vi "rx.vi"() -> ()   [LabVIEW 2020]
panel:
  out "array":i32[](array[numeric])
  out "read buffer":string
  in  "Serial Init":T1={"Puerto Serial"="", "baud rate (9600)"=9600, "data bits (8)"=8, "parity (0:none)"=enum."None", "error in (no error)"={"status"=FALSE, "code"=0, "source"=""}, "stop bits (10: 1 bit)"=10, "flow control (0:none)"=0} {"flow control (0:none)" items=["None", "XON/XOFF", "RTS/CTS", "XON/XOFF & RTS/CTS", "DTR/DSR", "XON/XOFF & DTR/DSR"]; "stop bits (10: 1 bit)" items=["1.0"=10, "1.5"=15, "2.0"=20]; "data bits (8)" min=5 max=8 step=1}
  in  "stop":bool
  # "Recepcion Serial"
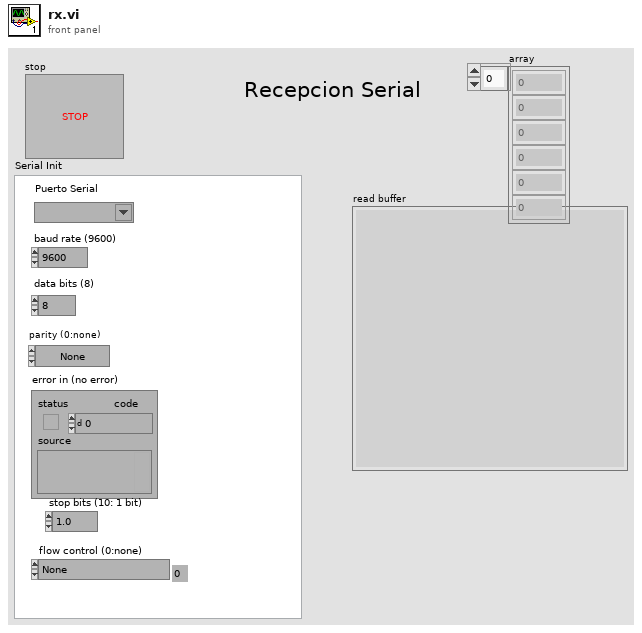
[diagram p1: front panel]
types:
  T1 = cluster{"Puerto Serial":refnum<visa-resource-name>, "baud rate (9600)":u32, "data bits (8)":u16, "parity (0:none)":enum16{"None", "Odd", "Even", "Mark", "Space"}, "error in (no error)":errorcluster, "stop bits (10: 1 bit)":u16, "flow control (0:none)":u16}
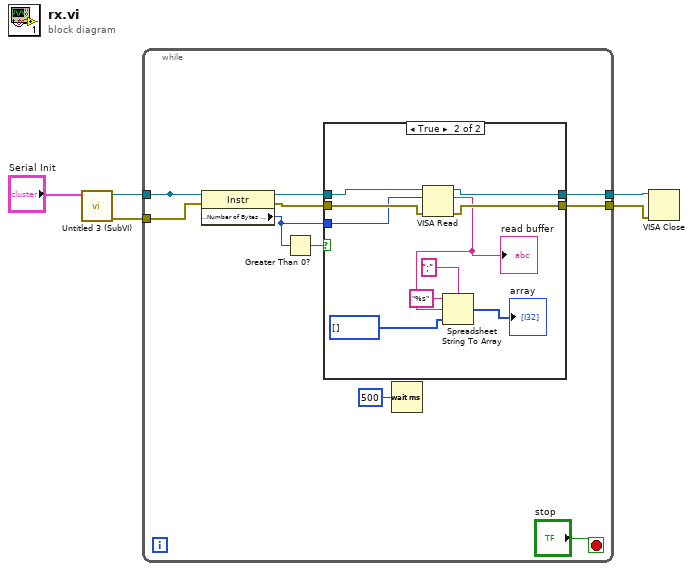
[diagram p0: block diagram]
diagram:
  n1 = call "Untitled 3 (SubVI).vi"("Serial Init"="Serial Init") -> ("error out"=w3:errorcluster, "VISA Refnum out"=w4:refnum<visa-resource-name>)  [unwired: 9 in]
  n2 = while {
    tunnel: [w14] -> _
    tunnel: w4 -> [w14]
    tunnel: w3 -> [w13]
    tunnel: [w10] -> w2
    tunnel: [w8] -> w1
    stop <- "stop" stop-if-true
    n3 = property class="Instr"(reference=w14, error in=w13) -> (reference out=w9:refnum<visa-resource-name>, error out=w7:errorcluster, "Serial Settings:Number of Bytes at Serial Port"=w6:u32)
    n4 = Greater Than 0?(x=w6) -> (x > 0?=w11:bool)
    n5 = case shown="True" w11 {
      tunnel: [w17 w24] -> w10
      tunnel: w9 -> [w17 w27]
      tunnel: [w16 w23] -> w8
      tunnel: w7 -> [w16 w26]
      tunnel: w6 -> [_ w25]
      frame False {
      }
      frame True {
        n6 = VISA Read(VISA resource name=w27, byte count=w25, error in (no error)=w26) -> (VISA resource name out=w24:refnum<visa-resource-name>, read buffer=w21:string, error out=w23:errorcluster)  [unwired: 1 out]
        "read buffer" <- w21
        n7 = Spreadsheet String To Array(delimiter (Tab)=";", format string="%s", spreadsheet string=w21, array type (2D Dbl)=i32[] []) -> (array=→"array":i32[])
      }
    }
    n8 = Wait (ms)(milliseconds to wait=u32 500) -> ()  [unwired: 1 out]
  }
  n9 = VISA Close(VISA resource name=w2, error in (no error)=w1) -> ()  [unwired: 1 out]
